vi "PDA_Exposure 1-D.vi"(7 "CCD GPIB Address":u16=1, 8 "error in":errorcluster, 11 "CCD Parameters":T1={"Exposure Time (s)"=0.2, "Offset"=0.0, "BkgrdCrct"=FALSE, "Shutter"=FALSE, "Mode"=enum."Regular", "Repetition"=4, "dt or s"=0.0} {"dt or s" format="%#.6f"; "Repetition" min=1; "Offset" format="%#.2f"; "Exposure Time (s)" min=0.02 max=6000.0 format="%#.2f"}) -> (0 "Error Out":errorcluster, 1 "#PixelOverflow":u32, 2 "PixelOverflow":bool, 3 "The Data":dbl[](array[numeric])=[1198.0, 1190.0, 1193.0, 1194.0, 1189.0, 1188.0, 1196.0, 1190.0, 1202.0, 1191.0, 1193.0, 1192.0, 1199.0, 1189.0, 1194.0, 1189.0, 1197.0, 1191.0, 1187.0, 1192.0, 1195.0, 1189.0, 1195.0, 1191.0, 1199.0, 1194.0, 1192.0, 1191.0, 1193.0, 1197.0, 1193.0, 1193.0, 1194.0, 1200.0, 1191.0, 1190.0, 1187.0, 1195.0, 1189.0, 1188.0, 1191.0, 1194.0, 1187.0, 1192.0, 1198.0, 1193.0, 1190.0, 1192.0, 1190.0, 1193.0, 1191.0, 1190.0, 1191.0, 1189.0, 1192.0, 1194.0, 1190.0, 1193.0, 1193.0, 1191.0, 1194.0, 1182.0, 1190.0, 1188.0, 1199.0, 1192.0, 1196.0, 1195.0, 1186.0, 1189.0, 1188.0, 1185.0, 1194.0, 1187.0, 1193.0, 1194.0, 1190.0, 1189.0, 1189.0, 1187.0, 1196.0, 1195.0, 1191.0, 1197.0, 1192.0, 1200.0, 1187.0, 1194.0, 1189.0, 1193.0, 1195.0, 1196.0, 1186.0, 1192.0, 1190.0, 1194.0, 1194.0, 1190.0, 1191.0, 1193.0, 1197.0, 1197.0, 1185.0, 1199.0, 1190.0, 1195.0, 1196.0, 1184.0, 1193.0, 1193.0, 1193.0, 1191.0, 1189.0, 1190.0, 1199.0, 1193.0, 1191.0, 1194.0, 1191.0, 1192.0, 1186.0, 1190.0, 1194.0, 1189.0, 1194.0, 1190.0, 1191.0, 1192.0, 1192.0, 1196.0, 1192.0, 1192.0, 1189.0, 1193.0, 1198.0, 1186.0, 1191.0, 1193.0, 1187.0, 1194.0, 1190.0, 1190.0, 1191.0, 1189.0, 1194.0, 1195.0, 1189.0, 1192.0, 1185.0, 1193.0, 1192.0, 1192.0, 1189.0, 1191.0, 1191.0, 1190.0, 1196.0, 1194.0, 1193.0, 1191.0, 1189.0, 1191.0, 1196.0, 1192.0, 1192.0, 1189.0, 1196.0, 1191.0, 1193.0, 1192.0, 1188.0, 1190.0, 1194.0, 1192.0, 1185.0, 1191.0, 1194.0, 1191.0, 1189.0, 1195.0, 1192.0, 1196.0, 1190.0, 1193.0, 1191.0, 1189.0, 1194.0, 1195.0, 1191.0, 1187.0, 1190.0, 1196.0, 1196.0, 1192.0, 1197.0, 1191.0, 1189.0, 1192.0, 1192.0, 1200.0, 1192.0, 1193.0, 1190.0, 1192.0, 1187.0, 1198.0, 1186.0, 1196.0, 1201.0, 1199.0, 1200.0, 1191.0, 1196.0, 1200.0, 1192.0, 1191.0, 1193.0, 1185.0, 1192.0, 1194.0, 1186.0, 1190.0, 1188.0, 1189.0, 1201.0, 1197.0, 1191.0, 1194.0, 1193.0, 1194.0, 1195.0, 1198.0, 1200.0, 1192.0, 1192.0, 1193.0, 1193.0, 1195.0, 1187.0, 1193.0, 1192.0, 1187.0, 1189.0, 1186.0, 1191.0, 1197.0, 1191.0, 1200.0, 1194.0, 1192.0, 1187.0, 1196.0, 1191.0, 1191.0, 1196.0, 1187.0, 1190.0, 1193.0, 1189.0, 1193.0, 1190.0, 1188.0, 1188.0, 1190.0, 1197.0, 1188.0, 1191.0, 1195.0, 1188.0, 1191.0, 1188.0, 1194.0, 1193.0, 1187.0, 1200.0, 1192.0, 1197.0, 1190.0, 1196.0, 1200.0, 1191.0, 1189.0, 1193.0, 1189.0, 1186.0, 1196.0, 1185.0, 1198.0, 1195.0, 1186.0, 1191.0, 1197.0, 1191.0, 1193.0, 1195.0, 1193.0, 1191.0, 1198.0, 1189.0, 1183.0, 1200.0, 1197.0, 1192.0, 1192.0, 1192.0, 1196.0, 1191.0, 1190.0, 1194.0, 1188.0, 1198.0, 1193.0, 1195.0, 1190.0, 1187.0, 1192.0, 1191.0, 1195.0, 1188.0, 1190.0, 1191.0, 1187.0, 1189.0, 1185.0, 1189.0, 1196.0, 1198.0, 1191.0, 1190.0, 1196.0, 1197.0, 1193.0, 1187.0, 1186.0, 1195.0, 1191.0, 1193.0, 1192.0, 1196.0, 1190.0, 1192.0, 1192.0, 1192.0, 1190.0, 1195.0, 1192.0, 1191.0, 1193.0, 1197.0, 1184.0, 1190.0, 1188.0, 1192.0, 1194.0, 1190.0, 1193.0, 1195.0, 1195.0, 1194.0, 1189.0, 1193.0, 1191.0, 1194.0, 1186.0, 1189.0, 1192.0, 1191.0, 1182.0, 1190.0, 1197.0, 1194.0, 1188.0, 1193.0, 1191.0, 1186.0, 1194.0, 1197.0, 1193.0, 1191.0, 1187.0, 1194.0, 1194.0, 1191.0, 1189.0, 1195.0, 1194.0, 1189.0, 1196.0, 1187.0, 1186.0, 1192.0, 1194.0, 1196.0, 1191.0, 1193.0, 1191.0, 1188.0, 1190.0, 1199.0, 1198.0, 1196.0, 1196.0, 1190.0, 1194.0, 1191.0, 1194.0, 1187.0, 1195.0, 1190.0, 1194.0, 1196.0, 1194.0, 1189.0, 1193.0, 1189.0, 1194.0, 1189.0, 1195.0, 1192.0, 1194.0, 1193.0, 1191.0, 1197.0, 1187.0, 1189.0, 1189.0, 1188.0, 1197.0, 1192.0, 1189.0, 1193.0, 1194.0, 1183.0, 1202.0, 1187.0, 1192.0, 1184.0, 1188.0, 1186.0, 1193.0, 1189.0, 1195.0, 1189.0, 1193.0, 1197.0, 1189.0, 1194.0, 1191.0, 1194.0, 1192.0, 1191.0, 1191.0, 1196.0, 1194.0, 1190.0, 1193.0, 1192.0, 1195.0, 1197.0, 1198.0, 1193.0, 1202.0, 1196.0, 1194.0, 1194.0, 1190.0, 1193.0, 1190.0, 1195.0, 1192.0, 1187.0, 1194.0, 1197.0, 1190.0, 1194.0, 1189.0, 1198.0, 1192.0, 1191.0, 1192.0, 1192.0, 1191.0, 1191.0, 1193.0, 1191.0, 1191.0, 1198.0, 1186.0, 1192.0, 1185.0, 1185.0, 1188.0, 1194.0, 1196.0, 1194.0, 1195.0, 1190.0, 1194.0, 1191.0, 1190.0, 1195.0, 1191.0, 1191.0, 1195.0, 1192.0, 1194.0, 1201.0, 1187.0, 1191.0, 1195.0, 1187.0, 1192.0, 1192.0, 1193.0, 1200.0, 1188.0, 1189.0, 1189.0, 1197.0, 1189.0, 1188.0, 1197.0, 1195.0, 1191.0, 1189.0, 1190.0, 1195.0, 1189.0, 1191.0, 1194.0, 1186.0, 1192.0, 1190.0, 1191.0, 1188.0, 1195.0, 1192.0, 1191.0, 1191.0, 1199.0, 1190.0, 1190.0, 1190.0, 1192.0, 1187.0, 1193.0, 1197.0, 1197.0, 1186.0, 1193.0, 1189.0, 1192.0, 1197.0, 1184.0, 1187.0, 1188.0, 1192.0, 1192.0, 1192.0, 1189.0, 1192.0, 1190.0, 1194.0, 1191.0, 1186.0, 1196.0, 1194.0, 1189.0, 1193.0, 1191.0, 1186.0, 1189.0, 1193.0, 1195.0, 1196.0, 1197.0, 1199.0, 1194.0, 1190.0, 1193.0, 1194.0, 1190.0, 1198.0, 1196.0, 1194.0, 1195.0, 1194.0, 1184.0, 1188.0, 1195.0, 1197.0, 1190.0, 1194.0, 1190.0, 1191.0, 1195.0, 1198.0, 1188.0, 1193.0, 1194.0, 1195.0, 1198.0, 1195.0, 1191.0, 1197.0, 1192.0, 1198.0, 1190.0, 1196.0, 1191.0, 1194.0, 1188.0, 1189.0, 1198.0, 1192.0, 1198.0, 1195.0, 1185.0, 1191.0, 1193.0, 1192.0, 1197.0, 1195.0, 1195.0, 1195.0, 1193.0, 1190.0, 1190.0, 1190.0, 1198.0, 1195.0, 1191.0, 1194.0, 1190.0, 1190.0, 1194.0, 1194.0, 1195.0, 1192.0, 1190.0, 1194.0, 1195.0, 1192.0, 1192.0, 1194.0, 1189.0, 1192.0, 1193.0, 1188.0, 1194.0, 1195.0, 1196.0, 1193.0, 1192.0, 1201.0, 1191.0, 1198.0, 1197.0, 1191.0, 1192.0, 1191.0, 1194.0, 1193.0, 1188.0, 1192.0, 1189.0, 1183.0, 1189.0, 1190.0, 1192.0, 1189.0, 1196.0, 1193.0, 1197.0, 1185.0, 1193.0, 1189.0, 1191.0, 1196.0, 1195.0, 1193.0, 1193.0, 1191.0, 1189.0, 1193.0, 1192.0, 1192.0, 1192.0, 1190.0, 1191.0, 1193.0, 1193.0, 1197.0, 1195.0, 1189.0, 1193.0, 1188.0, 1194.0, 1197.0, 1194.0, 1195.0, 1196.0, 1190.0, 1194.0, 1188.0, 1197.0, 1195.0, 1191.0, 1195.0, 1192.0, 1194.0, 1188.0, 1190.0, 1197.0, 1197.0, 1191.0, 1187.0, 1197.0, 1191.0, 1193.0, 1188.0, 1191.0, 1194.0, 1193.0, 1195.0, 1192.0, 1195.0, 1189.0, 1193.0, 1193.0, 1195.0, 1190.0, 1192.0, 1196.0, 1188.0, 1187.0, 1193.0, 1192.0, 1192.0, 1194.0, 1185.0, 1199.0, 1190.0, 1193.0, 1191.0, 1198.0, 1189.0, 1190.0, 1191.0, 1190.0, 1193.0, 1195.0, 1186.0, 1190.0, 1193.0, 1191.0, 1189.0, 1197.0, 1193.0, 1198.0, 1190.0, 1192.0, 1193.0, 1191.0, 1196.0, 1193.0, 1196.0, 1190.0, 1190.0, 1198.0, 1192.0, 1199.0, 1198.0, 1190.0, 1191.0, 1191.0, 1196.0, 1190.0, 1196.0, 1195.0, 1191.0, 1196.0, 1195.0, 1193.0, 1190.0, 1190.0, 1195.0, 1193.0, 1187.0, 1197.0, 1185.0, 1191.0, 1189.0, 1191.0, 1193.0, 1192.0, 1188.0, 1196.0, 1193.0, 1191.0, 1193.0, 1193.0, 1190.0, 1192.0, 1192.0, 1192.0, 1195.0, 1191.0, 1195.0, 1189.0, 1189.0, 1191.0, 1191.0, 1185.0, 1192.0, 1191.0, 1193.0, 1201.0, 1199.0, 1197.0, 1206.0, 1201.0, 1207.0, 1200.0, 1198.0, 1195.0, 1188.0, 1194.0, 1186.0, 1190.0, 1197.0, 1188.0, 1193.0, 1196.0, 1193.0, 1192.0, 1192.0, 1188.0, 1196.0, 1186.0, 1193.0, 1194.0, 1188.0, 1190.0, 1190.0, 1192.0, 1190.0, 1191.0, 1191.0, 1200.0, 1192.0, 1199.0, 1193.0, 1190.0, 1190.0, 1199.0, 1187.0, 1193.0, 1190.0, 1188.0, 1194.0, 1194.0, 1196.0, 1194.0, 1195.0, 1190.0, 1187.0, 1187.0, 1196.0, 1193.0, 1199.0, 1190.0, 1193.0, 1193.0, 1191.0, 1198.0, 1192.0, 1193.0, 1192.0, 1193.0, 1189.0, 1189.0, 1197.0, 1189.0, 1194.0, 1193.0, 1192.0, 1185.0, 1198.0, 1193.0, 1189.0, 1192.0, 1193.0, 1196.0, 1190.0, 1195.0, 1189.0, 1196.0, 1198.0, 1190.0, 1191.0, 1193.0, 1186.0, 1189.0, 1195.0, 1188.0, 1197.0, 1188.0, 1191.0, 1185.0, 1190.0, 1193.0, 1188.0, 1198.0, 1192.0, 1193.0, 1194.0, 1194.0, 1189.0, 1184.0, 1193.0, 1199.0, 1193.0, 1192.0, 1193.0, 1190.0, 1196.0, 1191.0, 1192.0, 1189.0, 1194.0, 1188.0, 1189.0, 1190.0, 1190.0, 1192.0, 1195.0, 1188.0, 1190.0, 1192.0, 1189.0, 1197.0, 1192.0, 1194.0, 1187.0, 1196.0, 1192.0, 1194.0, 1185.0, 1187.0, 1187.0, 1191.0, 1195.0, 1190.0, 1186.0, 1183.0, 1194.0, 1194.0, 1192.0, 1192.0, 1188.0, 1193.0, 1195.0, 1189.0, 1190.0, 1191.0, 1192.0, 1196.0, 1186.0, 1195.0, 1191.0, 1185.0, 1191.0, 1187.0, 1190.0, 1188.0, 1189.0, 1187.0, 1196.0, 1191.0, 1190.0, 1191.0, 1190.0, 1196.0, 1195.0, 1186.0, 1187.0, 1187.0, 1188.0, 1194.0, 1192.0, 1192.0, 1192.0, 1189.0, 1192.0, 1191.0, 1188.0, 1188.0, 1187.0, 1187.0, 1190.0, 1186.0, 1191.0, 1195.0, 1192.0, 1196.0, 1193.0, 1192.0, 1191.0, 1189.0, 1187.0, 1193.0, 1188.0, 1189.0, 1194.0, 1191.0, 1185.0, 1193.0, 1191.0, 1196.0, 1196.0, 1199.0, 1195.0, 1211.0] format="%.2f", 5 "Exposuretime (s) out":dbl format="%.2f")   [LabVIEW 2024]
uses:
  Globals and TypeDefs/Type Definitions.llb/CCDParameter.ctt
  Globals and TypeDefs/gDetector.vi
panel:
  out "Shot #":i32
  out "Repetition":u8=4 min=4
  out "Array Length":i32=1024
  out "Plot":dbl[][](graph)
  # "of"
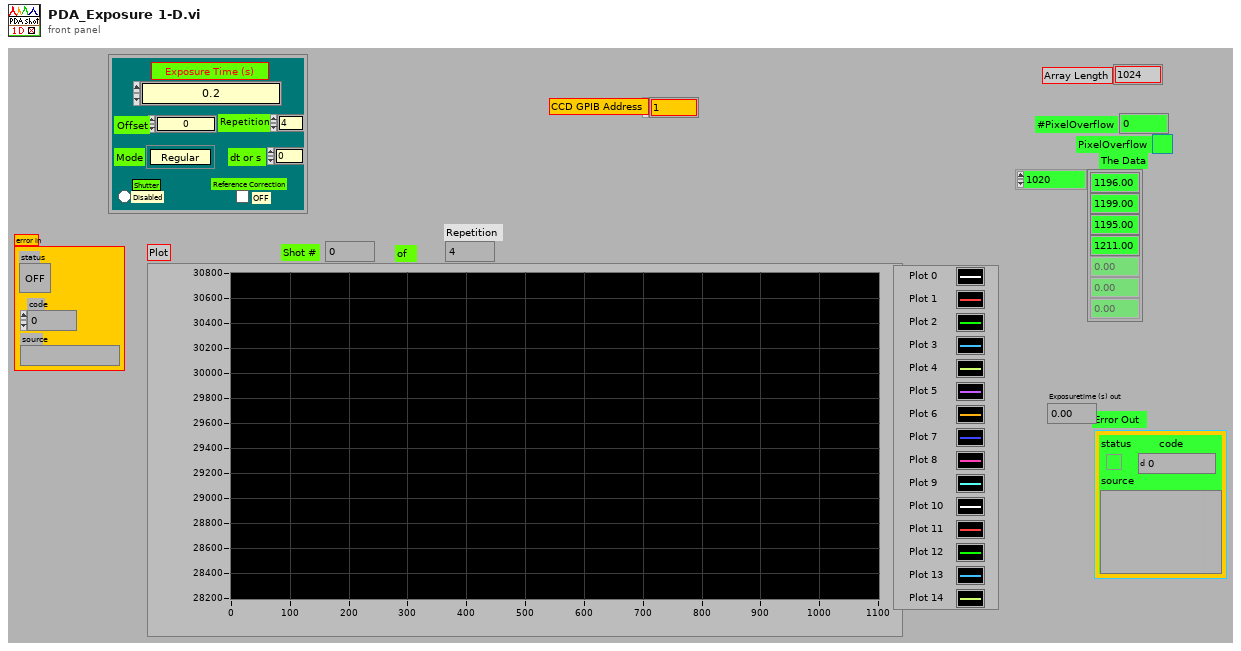
[diagram p1: front panel]
types:
  T1 = typedef "CCDParameter.ctt" = cluster{"Exposure Time (s)":dbl, "Offset":dbl, "BkgrdCrct":bool, "Shutter":bool, "Mode":enum8{"Regular", "OverExp Cor", "SpikeRemove", "ForCalibration"}, "Repetition":u16, "dt or s":dbl}
  T2 = enum8{"Regular", "OverExp Cor", "SpikeRemove", "ForCalibration"}
  T3 = cluster{"Exposure (ms)":u32, "Interval (ms)":u32, "Flush Count":i32, "Trigger":u16}
  T4 = enum16{"End", "Init", "Reset", "SetAcqParameter", "SetArea", "Start Acquisition", "Busy Status Poll", "Read", "Stop"}
  T5 = enum16{"End", "Init", "Reset", "SetAcqParameter", "SetArea", "AcqData"}
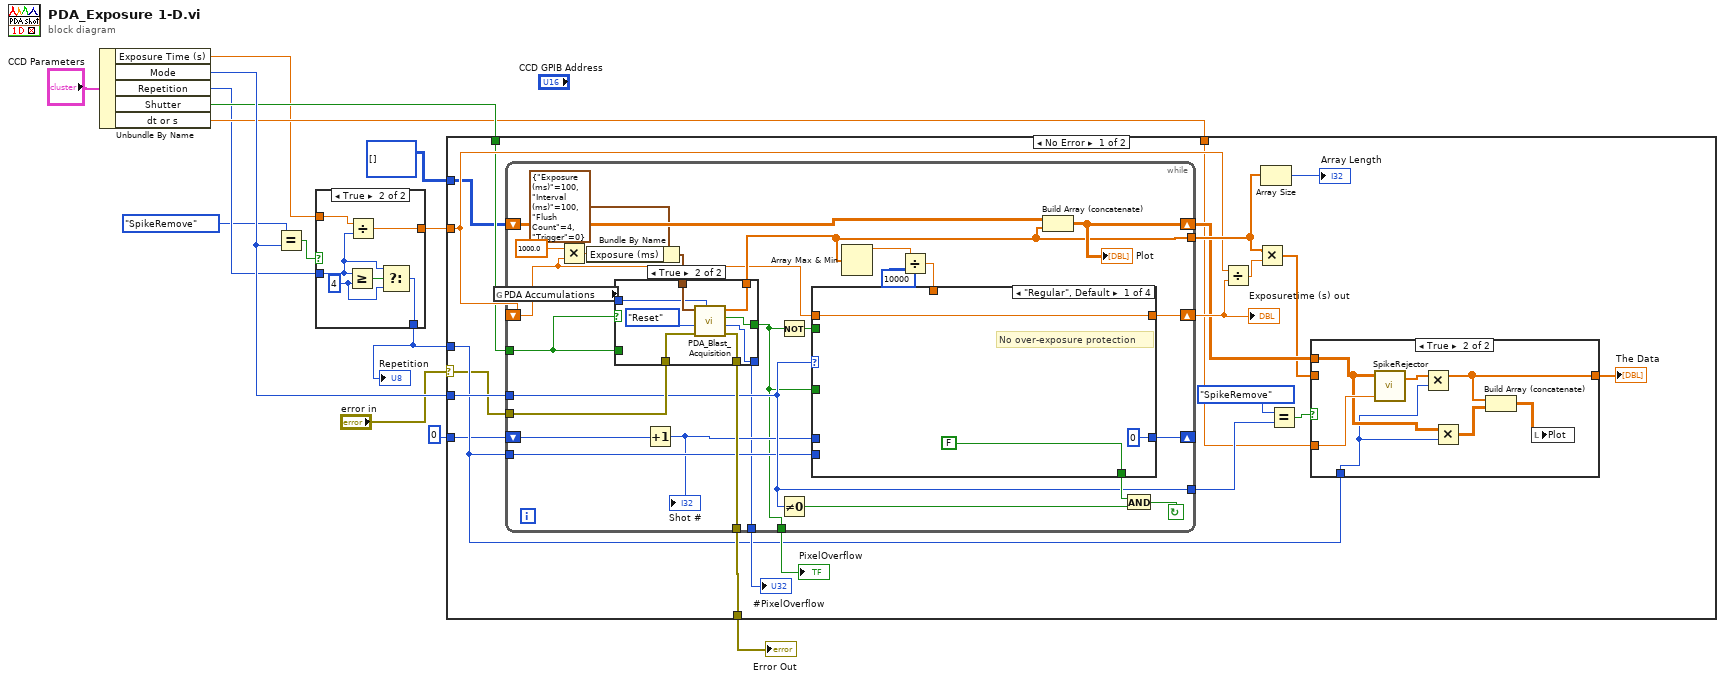
[diagram p0: block diagram]
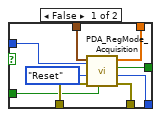
[diagram p4: hidden frame]
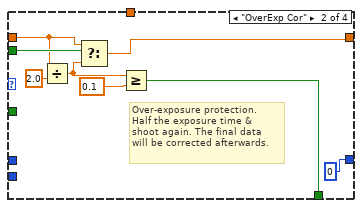
[diagram p5: hidden frame]
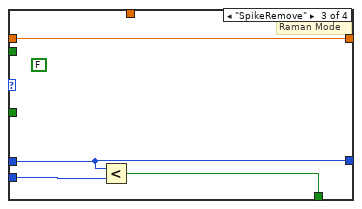
[diagram p6: hidden frame]
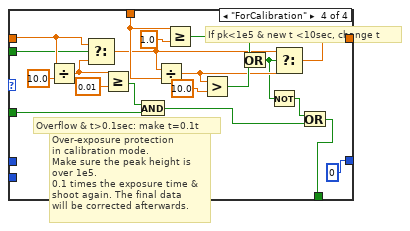
[diagram p7: hidden frame]
diagram:
  n1 = Unbundle By Name("CCD Parameters") -> ("Exposure Time (s)"=w4:dbl, "Mode"=w10:T2, "Repetition"=w7:u16, "Shutter"=w9:bool, "dt or s"=w8:dbl)
  n2 = Equal?(x=T2."SpikeRemove", y=w10) -> (x = y?=w13:bool)
  n3 = case shown="True" w13 {
    tunnel: w4 -> [w16 w22]
    tunnel: w7 -> [w15 w19]
    tunnel: [w16 w21] -> w12
    tunnel: [w15 w17] -> w6
    frame False {
    }
    frame True {
      w18 = u8 4 ("y")
      n4 = Greater Or Equal?(x=w19, y=w18) -> (x >= y?=w20:bool)
      n5 = Divide(x=w22, y=w19) -> (x/y=w21:dbl)
      n6 = Select(t=w19, s=w20, f=w18) -> (s? t:f=w17:u16)
    }
  }
  "Repetition" <- w6
  n7 = case shown="No Error" "error in" {
    selector: "error in" -> [w23 w131]
    tunnel: [w37 w131] -> w14
    tunnel: w10 -> [w31 _]
    tunnel: w6 -> [w29 _]
    tunnel: w12 -> [w30 _]
    tunnel: w9 -> [w28 _]
    tunnel: w8 -> [w27 _]
    tunnel: i32[][] [] -> [w25 _]
    tunnel: 0 -> [w24 _]
    frame No Error {
      n8 = while {
        tunnel: [w61] -> w38
        tunnel: [w60] -> w42
        tunnel: [w59] -> w43
        tunnel: [w69] -> w37
        shift-left: w30 -> [w55]
        shift-right: [w70] -> w41
        tunnel: w23 -> [w78]
        tunnel: w28 -> [w53]
        shift-right: [w68] -> _
        shift-left: w24 -> [w63]
        shift-right: [w66] -> w34
        shift-left: w25 -> [w67]
        tunnel: [w65] -> w36
        tunnel: w31 -> [w65]
        tunnel: w29 -> [w64]
        stop <- w77 continue-if-true
        n9 = global read "gDetector.vi" "PDA Accumulations"() -> (w52:i32)
        n10 = Multiply(x=1000.0, y=w55) -> (x*y=w58:dbl)
        n11 = Bundle By Name(cluster=T3 {"Exposure (ms)"=100, "Interval (ms)"=100, "Flush Count"=4, "Trigger"=0} ("Acquisition Parameters"), "Exposure (ms)"=w58) -> (w54:T3)
        n12 = case shown="True" w53 {
          tunnel: w78 -> [w87 w94]
          tunnel: [w86 w93] -> w69
          tunnel: [w85 w92] -> w61
          tunnel: [w84 w91] -> w60
          tunnel: [w83 w90] -> w59
          tunnel: w53 -> [w81 _]
          tunnel: w54 -> [w80 w95]
          tunnel: w52 -> [w79 w88]
          frame False {
            n13 = call "PDA_RegMode_Acquisition.vi"("Shutter"=w81, "error in"=w87, "StartIng Mode"=T4."Reset", "Number of Cycles"=w79, "Acquisition Parameters"=w80) -> ("error out"=w86:errorcluster, "# Pixel Overflow"=w83:i32, "PDA Overflow"=w84:bool, "Output Array"=w85:dbl[])
          }
          frame True {
            n14 = call "PDA_Blast_Acquisition.vi"("Number of Accumulations"=w88, "error in"=w94, "StartIng Mode"=T5."Reset", "Acquisition Parameters"=w95) -> ("error out"=w93:errorcluster, "Pixel Overflow"=w90:i32, "PDA Overflow"=w91:bool, "Final Data Array"=w92:dbl[])  [unwired: 2 in]
          }
        }
        n15 = Increment(x=w63) -> (x+1=w62:i32)
        "Shot #" <- w62
        n16 = Not(x=w60) -> (.not. x?=w74:bool)
        n17 = Not Equal To 0?(x=w65) -> (x != 0?=w76:bool)
        n18 = Array Max & Min(array=w61) -> (max value=w73:dbl)  [unwired: 3 out]
        n19 = Divide(x=w73, y=10000) -> (x/y=w71:dbl)
        n20 = case shown="\"Regular\", Default" w65 {
          tunnel: [w98 w100 w110 w118] -> w70
          tunnel: w55 -> [w98 w102 w110 w127]
          tunnel: [FALSE w104 w109 w116] -> w75
          tunnel: w74 -> [_ w103 _ w126]
          tunnel: w71 -> [_ _ _ w124]
          tunnel: [0 0 w107 0] -> w68
          tunnel: w60 -> [_ _ _ w114]
          tunnel: w64 -> [_ _ w108 _]
          tunnel: w62 -> [_ _ w107 _]
          frame "Regular", Default {
            # "No over-exposure protection"
          }
          frame "OverExp Cor" {
            # "Over-exposure protection.\nHalf the exposure time &\nshoot again. The final data\nwill be corrected afterwards."
            n21 = Divide(x=w102, y=2.0) -> (x/y=w101:dbl)
            n22 = Select(t=w102, s=w103, f=w101) -> (s? t:f=w100:dbl)
            n23 = Greater Or Equal?(x=w101, y=0.1) -> (x >= y?=w104:bool)
          }
          frame "SpikeRemove" {
            (unwired) FALSE
            # "Raman Mode"
            n24 = Less?(x=w107, y=w108) -> (x < y?=w109:bool)
          }
          frame "ForCalibration" {
            # "If pk<1e5 & new t <10sec, change t"
            # "Overflow & t>0.1sec: make t=0.1t"
            # "Over-exposure protection\nin calibration mode. \nMake sure the peak height is \nover 1e5.\n0.1 times the exposure time &\nshoot again. The final data\nwill be corrected afterwards."
            n25 = Divide(x=w127, y=10.0) -> (x/y=w128:dbl)
            n26 = Select(t=w127, s=w126, f=w128) -> (s? t:f=w120:dbl)
            n27 = Greater Or Equal?(x=w128, y=0.01) -> (x >= y?=w115:bool)
            n28 = And(x=w115, y=w114) -> (x .and. y?=w113:bool)
            n29 = Divide(x=w120, y=w124) -> (x/y=w119:dbl)
            n30 = Greater Or Equal?(x=w124, y=1.0) -> (x >= y?=w121:bool)
            n31 = Greater?(x=w119, y=10.0) -> (0:w122:bool)
            n32 = Or(x=w121, y=w122) -> (x .or. y?=w111:bool)
            n33 = Not(x=w111) -> (.not. x?=w112:bool)
            n34 = Select(t=w120, s=w111, f=w119) -> (s? t:f=w118:dbl)
            n35 = Or(x=w112, y=w113) -> (x .or. y?=w116:bool)
          }
        }
        n36 = Build Array (concatenate)(w67, w61) -> (w66:dbl[][])
        "Plot" <- w66
        n37 = And(x=w75, y=w76) -> (x .and. y?=w77:bool)
      }
      "PixelOverflow" <- w42
      "#PixelOverflow" <- w43
      "Exposuretime (s) out" <- w41
      n38 = Divide(x=w30, y=w41) -> (x/y=w40:dbl)
      n39 = Multiply(x=w38, y=w40) -> (x*y=w33:dbl[])
      n40 = Array Size(array=w38) -> (size(s)=→"Array Length":i32)
      n41 = Equal?(x=T2."SpikeRemove", y=w36) -> (x = y?=w35:bool)
      n42 = case shown="True" w35 {
        tunnel: w27 -> [_ w51]
        tunnel: w34 -> [_ w47]
        tunnel: w33 -> [w44 _]
        tunnel: [w44 w49] -> w32
        tunnel: w29 -> [_ w46]
        frame False {
        }
        frame True {
          n43 = call "SpikeRejector.vi"("SigmaFactor"=w51, "Input Array"=w47) -> ("Final Array"=w50:dbl[])  [unwired: 2 in, 1 out]
          n44 = Multiply(x=w50, y=w46) -> (x*y=w49:dbl[])
          n45 = Multiply(x=w47, y=w46) -> (x*y=w45:dbl[][])
          n46 = Build Array (concatenate)(w49, w45) -> (w48:dbl[][])
          n47 = local write "Plot"(w48) -> ()
        }
      }
      "The Data" <- w32
    }
    frame Error {
    }
  }
  "Error Out" <- w14
